vi "Tosca-Adjust Laser PWM.vi"(0 "SigMan in":refnum<class "SignalManager.lvclass">, 11 "error in (no error)":errorcluster) -> (4 "SigMan out":refnum<class "SignalManager.lvclass">, 15 "error out":errorcluster)   [LabVIEW 2020]
uses:
  epl-vi-lib/Signal Synthesis VIs/4th Generation/Classes/SignalManager/SignalManager.lvclass
  epl-vi-lib/Signal Synthesis VIs/4th Generation/Classes/Level/LevelUnits.ctl
  epl-vi-lib/Signal Synthesis VIs/4th Generation/Classes/Channel/Channel.lvclass/Channel.ctl
  epl-vi-lib/Signal Synthesis VIs/4th Generation/Classes/Level/Level.lvclass/Level.ctl
  epl-vi-lib/Signal Synthesis VIs/4th Generation/Classes/Waveforms/Pulse Train/Pulse Train.lvclass
  D:/Experiment VIs/Signal Synthesis VIs/4th Generation/Classes/Waveforms/Waveform/Waveform.lvclass
  epl-vi-lib/Signal Synthesis VIs/4th Generation/Classes/Channel/Write Waveform.vi
  epl-vi-lib/Signal Synthesis VIs/4th Generation/Classes/Channel/Write Level.vi
  epl-vi-lib/Signal Synthesis VIs/4th Generation/Classes/Channel/Read Waveform.vi
  epl-vi-lib/Signal Synthesis VIs/4th Generation/Classes/Channel/Read Level.vi
  epl-vi-lib/Signal Synthesis VIs/4th Generation/Classes/Level/Read Units.vi
  epl-vi-lib/Signal Synthesis VIs/4th Generation/Classes/Waveforms/Waveform/Waveform.lvclass
  D:/Experiment VIs/Koop/KObject Class/KObject.lvclass
  epl-vi-lib/Signal Synthesis VIs/4th Generation/Classes/Level/Level.lvclass
  epl-vi-lib/Koop/KObject Class/KObject.lvclass
  epl-vi-lib/Signal Synthesis VIs/4th Generation/Classes/Channel/Channel.lvclass
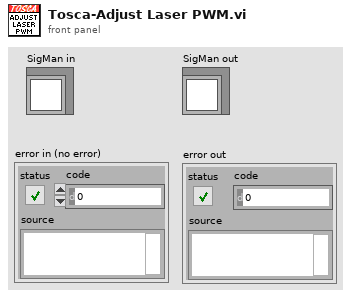
[diagram p1: front panel]
types:
  T1 = typedef "Level.lvclass/LevelUnits.ctl" = enum16{"dB atten", "dB SPL", "dB Vrms", "Volts", "dB mW", "mW", "dB HL", "dB SL"}
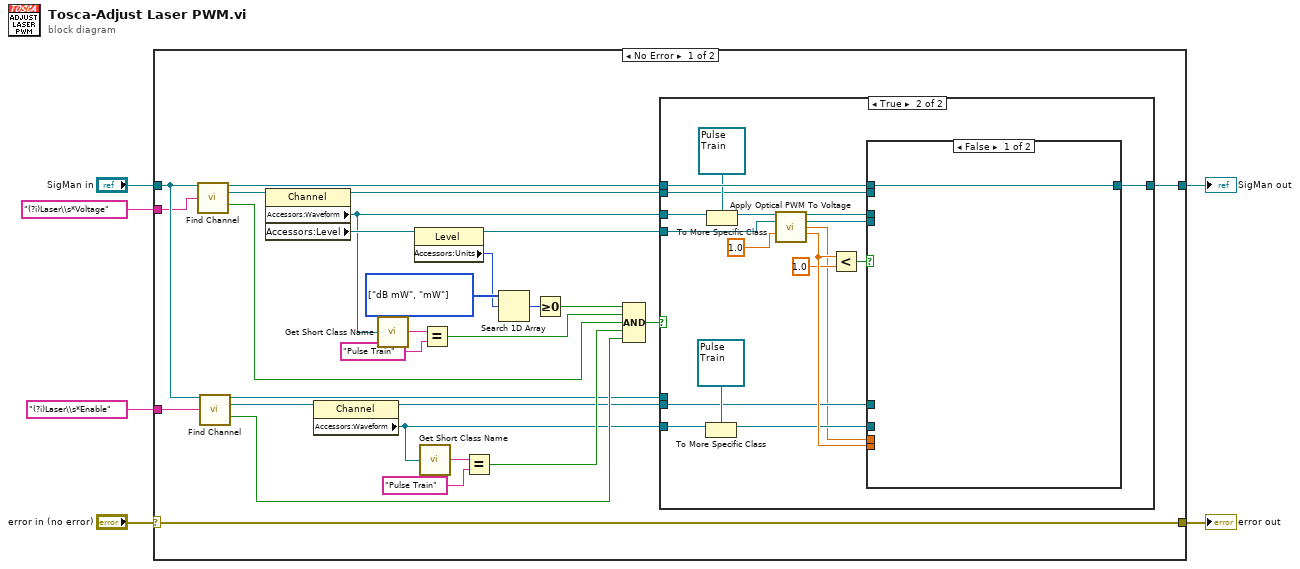
[diagram p0: block diagram]
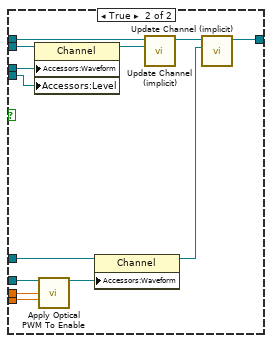
[diagram p3: hidden frame]
diagram:
  n1 = case shown="No Error" "error in (no error)" {
    selector: "error in (no error)" -> [w7 w68]
    tunnel: "SigMan in" -> [w27 w69]
    tunnel: "(?i)Laser\\s*Enable" ("regular expression") -> [w26 _]
    tunnel: "(?i)Laser\\s*Voltage" ("regular expression") -> [w25 _]
    tunnel: [w8 w69] -> w2
    tunnel: [w7 w68] -> w1
    frame No Error {
      w20 = T1[] [enum."dB mW", enum."mW"] items=["dB atten", "dB SPL", "dB Vrms", "Volts", "dB mW", "mW", "dB HL", "dB SL"] ("x")
      n2 = call "Find Channel.vi"("SigMan in"=w27, "regular expression"=w25) -> ("SigMan out"=w15:refnum<class "SignalManager.lvclass">, "Channel"=w21:refnum<class "Channel.lvclass">, "found"=w31:bool)  [unwired: 10 in, 1 out]
      n3 = call "Find Channel.vi"("SigMan in"=w27, "regular expression"=w26) -> ("SigMan out"=w22:refnum<class "SignalManager.lvclass">, "Channel"=w12:refnum<class "Channel.lvclass">, "found"=w23:bool)  [unwired: 10 in, 1 out]
      n4 = property class="Channel"(reference=w21) -> (reference out=w17:refnum<class "Channel.lvclass">, "Accessors:Waveform"=w13:refnum<class "Waveform.lvclass">, "Accessors:Level"=w14:refnum<class "Level.lvclass">)  [unwired: 1 in, 1 out]
      n5 = property class="Channel"(reference=w12) -> (reference out=w11:refnum<class "Channel.lvclass">, "Accessors:Waveform"=w10:refnum<class "Waveform.lvclass">)  [unwired: 1 in, 1 out]
      n6 = call "Get Short Class Name.vi"("KObject in"=w13) -> ("Class"=w34:string)  [unwired: 4 in]
      n7 = property class="Level"(reference=w14) -> (reference out=w9:refnum<class "Level.lvclass">, "Accessors:Units"=w16:T1)  [unwired: 1 in, 1 out]
      n8 = call "Get Short Class Name.vi"("KObject in"=w10) -> ("Class"=w29:string)  [unwired: 4 in]
      n9 = Equal?(x=w34, y="Pulse Train") -> (x = y?=w32:bool)
      n10 = Equal?(x=w29, y="Pulse Train") -> (x = y?=w24:bool)
      n11 = Search 1D Array(1D array=w20, element=w16) -> (index of element=w19:i32)  [unwired: 1 in]
      n12 = Greater Or Equal To 0?(x=w19) -> (x >= 0?=w18:bool)
      n13 = Compound Arithmetic op=AND(w18, w32, w31, w24, w23) -> (w30:bool)
      n14 = case shown="True" w30 {
        tunnel: w22 -> [_ _]
        tunnel: w17 -> [_ w47]
        tunnel: w15 -> [w35 w53]
        tunnel: [w35 w52] -> w8
        tunnel: w13 -> [_ w51]
        tunnel: w11 -> [_ w39]
        tunnel: w10 -> [_ w41]
        tunnel: w9 -> [_ w38]
        frame False {
        }
        frame True {
          n15 = To More Specific Class(target class=refnum<class "Pulse Train.lvclass"> refnum ("Pulse Train"), reference=w41) -> (specific class reference=w40:refnum<class "Pulse Train.lvclass">)  [unwired: 1 in, 1 out]
          n16 = To More Specific Class(target class=refnum<class "Pulse Train.lvclass"> refnum ("Pulse Train"), reference=w51) -> (specific class reference=w50:refnum<class "Pulse Train.lvclass">)  [unwired: 1 in, 1 out]
          n17 = call "Apply Optical PWM To Voltage.vi"("Pulse Train in"=w50, "Level in"=w38, "Min voltage"=1.0 ("multiplier")) -> ("Pulse Train out"=w48:refnum<class "Pulse Train.lvclass">, "Level out"=w37:refnum<class "Level.lvclass">, "Pulse width (us)"=w36:dbl, "PWM factor"=w44:dbl)  [unwired: 8 in, 1 out]
          n18 = Less?(x=w44, y=1.0) -> (x < y?=w45:bool)
          n19 = case shown="False" w45 {
            tunnel: w53 -> [w54 w67]
            tunnel: [w54 w58] -> w52
            tunnel: w48 -> [_ w66]
            tunnel: w47 -> [_ w65]
            tunnel: w44 -> [_ w62]
            tunnel: w40 -> [_ w63]
            tunnel: w39 -> [_ w61]
            tunnel: w37 -> [_ w56]
            tunnel: w36 -> [_ w55]
            frame False {
            }
            frame True {
              n20 = property class="Channel"(reference=w65, "Accessors:Waveform"=w66, "Accessors:Level"=w56) -> (reference out=w64:refnum<class "Channel.lvclass">)  [unwired: 1 in, 1 out]
              n21 = call "Apply Optical PWM To Enable.vi"("Pulse Train in"=w63, "Pulse width (us)"=w55, "PWM factor"=w62) -> ("Pulse Train out"=w60:refnum<class "Pulse Train.lvclass">)  [unwired: 11 in, 1 out]
              n22 = property class="Channel"(reference=w61, "Accessors:Waveform"=w60) -> (reference out=w57:refnum<class "Channel.lvclass">)  [unwired: 1 in, 1 out]
              n23 = call "Update Channel (implicit).vi"("Channel"=w64, "SignalManager in"=w67) -> ("SignalManager out"=w59:refnum<class "SignalManager.lvclass">)  [unwired: 8 in, 1 out]
              n24 = call "Update Channel (implicit).vi"("Channel"=w57, "SignalManager in"=w59) -> ("SignalManager out"=w58:refnum<class "SignalManager.lvclass">)  [unwired: 8 in, 1 out]
            }
          }
        }
      }
    }
    frame Error {
    }
  }
  "error out" <- w1
  "SigMan out" <- w2
